vi "mxwScript_Cmnd2Str_setTemplateRef.vi"(8 "error in (no error)":errorcluster, 11 "data":variant) -> (0 "error out":errorcluster, 3 "outputString":string)   [LabVIEW 2017]
uses:
  codeGenAPISupport.llb/cgAPI_mxwScript_DrpTmplt_TemplateRefData.ctl
  codeGenAPISupport.llb/cgAPI_mxwScript_DrpTmplt_TemplateRefType.ctl
  codeGenAPISupport.llb/cgAPI_mxwScript_DrpTmplt_ReferencePosition.ctl
  codeGenAPISupport.llb/cgAPI_mxwScript_DrpTmplt_TerminalData.ctl
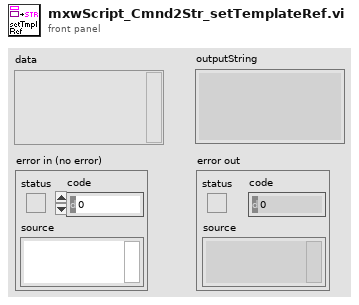
[diagram p1: front panel]
types:
  T1 = typedef "cgAPI_mxwScript_DrpTmplt_TemplateRefData.ctl" = cluster{"type":T2, "refPosition":T3, "terminalData":T4}
  T2 = typedef "cgAPI_mxwScript_DrpTmplt_TemplateRefType.ctl" = enum16{"InputAverage", "Absolute", "Terminal"}
  T3 = typedef "cgAPI_mxwScript_DrpTmplt_ReferencePosition.ctl" = enum16{"TopLeft", "Top", "TopRight", "Left", "Middle", "Right", "BottomLeft", "Bottom", "BottomRight"}
  T4 = typedef "cgAPI_mxwScript_DrpTmplt_TerminalData.ctl" = cluster{"name":string, "termIsTag":bool, "referencePosition":T3}
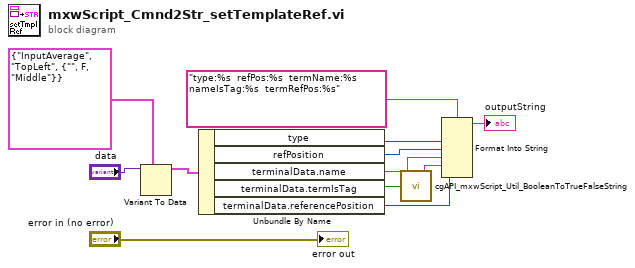
[diagram p0: block diagram]
diagram:
  n1 = Variant To Data(type=T1 {"type"=enum."InputAverage", "refPosition"=enum."TopLeft", "terminalData"={"name"="", "termIsTag"=FALSE, "referencePosition"=enum."Middle"}} ("targetRefData"), Variant="data") -> (data=w10:T1)  [unwired: 1 in, 1 out]
  n2 = Unbundle By Name(w10) -> ("type"=w8:T2, "refPosition"=w6:T3, "terminalData.name"=w3:string, "terminalData.termIsTag"=w2:bool, "terminalData.referencePosition"=w4:T3)
  n3 = call "cgAPI_mxwScript_Util_BooleanToTrueFalseString.vi"("boolean"=w2) -> ("TRUE/FALSE text"=w1:string)  [unwired: 4 out]
  n4 = Format Into String(format string="type:%s  refPos:%s  termName:%s  nameIsTag:%s  termRefPos:%s", w8, w6, w3, w1, w4) -> (resulting string=→"outputString":string)  [unwired: 2 in, 1 out]
  "error out" <- "error in (no error)"
